vi "Main_21b.vi"() -> ()   [LabVIEW 2020]
uses:
  ENUM_Operator.ctl
  <vilib>/Utility/miscctls.llb/LVMapReplaceAction.ctl
  Cluster 21b_Monkey Data.ctl
  Map21b_Monkey Data.ctl
panel:
  out "value":i64
  out "data":string
  out "Map 2":T1
  out "total":i32
  out "itteration":i32
  out "Map":T1
  out "Answer":i32
  in  "Puzzle":string="jntc: tzrz * jmgz\nchsl: rbmj + chpp\ntmjp: rlbw + prhj\nrllz: wrgr * jplq\nbttz: hslv + jsph\npbcg: frwf - vzrg\ngfhs: 4\nsglc: 8\nrqmt: 2\nfltv: 2\nzggp: thct * ddvm\ncqdj: 8\nmslt: gsnz + blhq\nmrqj: vzvz * sdnf\nbqfd: jtlf - hmfq\npgsr: 2\nbgmj: vhqn + nnrs\nqjgh: 2\nvbwn: 2\ndftr: 2\nrphr: tnjt + vwds\nwjqp: 3\njqvb: 11\ndjcv: rtzp + ltmf\npzfg: frcg + gwdc\nsbvb: zqvr / qbtm\nfhwn: tbjd + szcc\nwdrt: 3\nhplr: gtwd * jbss\nsvgc: lddn + czqc\ncmjg: 5\nmmvj: jlbq * zdcv\nfpmz: gzjs * lwdn\ndvht: 5\ncffj: hddd + qjrz\nqcvt: rlhd * ljqt\nswqg: bvnb * wrsz\nsbmb: 7\nzmph: 3\nvjcd: qplm + fvsm\nggwg: pdfh * pjtb\nmvnq: 2\nzjgh: hqpr + bbgs\ncwzv: wfzn * dwtq\nwswt: 17\nhslp: 2\nmsct: chtt * tcvm\nfrwt: jnts * qpsz\nhnvf: pbwq + bhzw\nznsz: 2\nwfbs: 5\ndgwc: 13\ngcwt: 3\ncrhj: pznp * vcvv\npqzd: jjsc * gjnr\nqfjf: 5\ntbjd: 6\nlglj: ghnb * jdzl\ncwfj: 9\nlvqr: nlgh + nqfp\nszfs: dwdn - mcjd\ntgjh: 4\nvccz: dgcb + pqbm\nnmvr: wwvn * rsdv\ntblc: 5\nbqdv: 9\nnsft: 3\nqgvr: bpzw * mgvr\njswp: 3\nqmbr: 5\nzdcv: tlnj + qsff\nqbns: tprb / qvzt\nlftn: fmbw * jzjp\nzngc: 4\nvqzd: hjmb / dspt\nbvdt: 3\ncpqr: 2\nclhj: 5\njnnp: 2\nmjhm: 16\nzzrp: qcrs + gtbj\ntgjj: rcsj * mwmr\nrfqb: ncnl + dwgd\nzhcb: gsng + gnhq\nbbsr: 3\ndpfm: 1\nmrmp: sgvw * cmdh\ngbwd: 18\nzhcs: 3\nhnrz: 2\nwwvn: 3\nhbth: dcwg + fjrb\nbsqw: bqfd + sncr\nqzpl: fqrd * gqlh\nchtt: 10\ndtqz: 4\nsjhh: 17\nwhhm: 4\nplqr: 1\nnbmb: bvtc - ngwv\nzgcs: 2\njzjp: 2\njbfs: 11\ncchn: dpgb + ptjg\nwgvf: slhc + gmnw\ndvrf: 2\nbhjn: 2\nvrms: tczg * rhlg\nplcs: 4\ngjcs: 7\nwdfz: slwr + nqlt\ndjfv: ncjg + dbmw\ngfbs: fsrz * cqgh\nhfwt: 2\ntcpv: jgjb + vwcm\nbmjq: cpwb + nmvw\nnrwh: 4\nfqrd: 6\ndwjj: 4\npjwh: lghd / cftw\nbrwh: sbzv * cmjg\nvpts: zqnn + hflj\nvqds: vgsm + pmnv\nznlq: bqgv + dhzl\nfcls: bvbj / qpfh\nrhvf: 19\nnqnw: 3\nmlfm: 4\ngzjq: 2\nzfln: pwqd * sbmd\nqqst: jfhc * qcvt\nzprj: 3\nrvmz: ntdt + zhjb\nlqdh: cgrj + lfls\nlnbf: rtfj * ghlw\nmwdb: 9\nrclm: 12\nqpsz: 14\nqthm: rrmz * tfhq\nfmbt: twzz * wchd\nfvpj: plgp * nmtc\nqfjl: 7\nvcwg: smsr * dmdl\npttw: 8\nhwqm: znmm + mhwn\ncrnl: tdvz * fqtj\nfzwp: 5\nswfd: tscb * hdgq\nnlgh: cgdh - vdch\ndbfp: 12\npzbr: qrzt * shjp\ngmbz: chqv * lhwn\ndmjp: 2\ncjcl: 4\nljbm: 2\ntjhg: svdh * svcm\nwztf: 5\nvpmw: thmn + mtvl\nnfqr: 3\ncdzs: pntb + ncbg\nmhtc: 3\nprrj: jvvr / mpzh\nnbqf: rtvl * lqdh\nbnvv: qdgh + tght\nnqdj: 4\njmgn: 2\ngbpb: dnch * cnjf\nrgth: hmdh + vchv\nlmvn: 13\nlslm: 4\nltzd: sgwp * cmng\nfsrz: 2\nzvgp: fwhj * pzgj\nlvhs: 5\nctvm: lfvt * vmmb\ndjvv: lzjn * rclm\ntgbp: vhgv + hjch\nsjwz: 3\nqcpj: 4\nmmgz: 3\nqglw: 3\nvlgr: 2\nvcgp: hhsq + jhzd\nzhzd: 2\ntmpn: 2\nhdcz: wjhs * bbgl\ntshl: jncw - hsdj\nchps: 4\nthwz: 9\nlbzf: nfgg - bmcs\nffmm: zhjp * rbvs\nwpql: htrh / zggd\nmrmf: 19\nwnwl: jdph * fwdq\nfhfq: pgqt + fbcc\ntscb: 3\njnwm: 10\nfjhr: nftz * brss\nnsgc: 3\ndplt: 7\nwstd: ltgp + rnrf\nhztd: 5\nvnjz: brnn * bcwv\nspbn: wnjz * wnql\njhvq: 13\nzvsq: 5\nhjlp: 2\nbslw: 1\ngzzf: qwzc * wfbs\njqqv: 2\nflnz: gpfs + fnnp\nrtcg: dbfd / pfsm\ngsnz: wfts + mbnv\nnlnn: 3\njvpc: fcbt + rphr\nbdvw: jtzh * tdmd\nlzqm: 6\njtzh: 2\ntlhl: 3\nhlpt: wvfm * ssls\nmfbr: tgbp * tdtb\nwsjg: qvww + qllf\nwsdf: 15\nrtgw: 11\nfwdq: 2\njdph: mqbs * ctzc\nmrtl: 2\nhfnd: srzl * fbcb\nrgrh: 7\nnltl: 11\npgns: zffq * pbbd\nmcpb: 9\njmtj: 17\nvhfz: 8\njqmf: 7\nfrbg: 20\nqqrz: 2\ntrmp: 18\nrhng: tdmm * phjw\njmll: 12\nvqjv: 3\ntdmd: zvff + zggr\nplvh: 16\nlgfr: 3\ngncb: 2\ngvmf: 3\nrlbw: 2\nhjch: bwwq * fdsm\nnlzl: hfnd * hlrh\ntfrj: 20\nrnrf: mrgm * vwhf\nnvmm: 1\nwgmz: rhcp / rlmn\nhpbq: 3\nqjfp: 3\npjqj: 10\ndwwh: 2\nqpmt: ssjf * bmrj\njmqm: hmlj + tfcl\ngzsw: 2\nwmgn: 4\ndstw: ptbp + qnrd\nvznm: qvvs * nsft\npczb: cdfz * ghbn\nbzdz: lslm + jsdw\nhlhg: jmll + mhrz\nfgdw: wtsj * fpbt\njbbg: 3\nhfbj: 7\nrzqq: wbgw * tzdd\nlhwn: 4\npndj: 5\nszws: 4\nfrwf: jcjg + jsnv\npjfc: rtcq / zfdr\njrqq: zvsm + qzhz\nsdfq: 3\nnvmn: znlq * ssql\nqzhf: 6\nhrrn: 20\nfgjt: 11\nzhlq: 4\nnfgg: dnfh - psls\npnrq: fbzq + lbqm\nspqg: 3\nblgg: 13\ntswl: mvmn * sqbn\nqsmp: 2\ndtdb: 3\njmjp: 3\nsprd: 2\nzgmr: 3\nmwpb: pqsg + ppsm\nsjld: 2\nmvhz: nslp / wmgn\nddsm: 2\nrqnr: rlfb + nrwh\nrsnc: spth - hqfs\ndwgj: 2\ntcdj: bttz * fmnh\nvpbh: lhjn / gmcq\nnpqv: dmqt * dstn\nqmwm: jsnt + jvzj\npvtq: 9\npvhz: tstp * ltdn\nthmn: 9\nchpc: mqws * rppc\ndwdn: ndgs * nlnn\nzzpb: bvqg + pjjh\nhpfn: 5\ndfqh: fpvz - hgtm\nwnbm: 2\nczjp: 3\njcsg: 2\ndvjh: rzqq + cpvv\nwdnd: sbvw * hlrj\nlgvh: 4\nlpbr: mbww + qsmp\nmgvn: ppgd + djvv\njjlt: 20\ntzrz: 3\ncqct: hbqd / dfcj\nqzsq: 6\ndqvj: rfnc + wqzg\nhvfp: hndj + cndw\nsgqv: 19\nsvdh: 2\ncrhl: cfsr / lwhh\npwgm: 9\npgmw: 7\nccvc: qmrn + twjr\nsvsl: bmws + qjqp\njzqs: 2\nrbmj: 13\nsgwp: 9\ntlbm: fvln * jjbr\nvcwc: mrbm + rvgm\nnpzj: nbmb / cmrn\nfvzd: mfjt + gtgn\nfjbh: 2\nhtrh: cjlc * gjrf\nhlfv: zszm * pzsz\npcvb: 2\nhdbc: zwbs - rndg\nqjdc: tmjp * pmsh\nrtfb: jppl / qpft\nbdln: 2\nqqzj: vrms * nvhp\nlbrd: 5\nchlh: vsgd + gqgq\nrlpp: mnmv + wtwr\nzdzr: jnwm + cndn\nsgqc: 3\nhdgq: 3\ndsms: jmtj * svqr\nrlcp: gjcs + lnmr\nszll: 2\nbhjg: 3\nnllp: 7\nptjg: mlfm * ptbv\njfhc: 2\nqsff: 4\ngcsg: 2\njgpp: rgsh + crjw\nqghb: rqjn / bnnv\nglwr: zphr * tnzz\nvvmr: 2\ndgcb: mpqs + snbz\nbsng: sjwz + rzzm\npbcq: wgrl + ccvc\nczwl: djjt + wspf\nbslv: jlff + nvzz\npznp: 2\ndtnv: cpgw - gpvb\nsdqw: 5\ngcnq: 2\ntpnh: 2\nzmnq: qglt / tgjw\nvwnz: 5\ncmms: jgpp + rdnh\nvzwn: 2\nhqpr: 12\nqjqp: hqsp * hwrg\ndgtj: wdzt * zcnc\nnwfw: 5\nhghn: 5\nqlfm: 3\nlgtd: mcgl / vdnj\nvnct: 2\nrqjn: jnjd + hdwc\nbpql: wgvf + pmpc\nbgrc: cglv - lmmt\nljrp: 1\ntvsj: 9\nfrzb: 2\nngnc: 1\nhhsq: 2\nqwcb: 6\nljcf: 19\nwrgm: 5\nzwbs: gvjr * gztn\nbhsl: 6\nbrpr: 2\nhfrs: 5\nwdmd: 2\nvsvn: 2\nzhmz: sfld + rhng\nddvm: spnl * mwdg\nvmlh: cwzs + wnwl\ncwzs: 4\ngwfg: 4\nsnhj: gfjq + jqmf\ncwmv: 5\nppvp: rtwl * wqvr\nbqdt: bcmg + lpsh\nqpft: 3\nbcwv: mhfj + mdpd\njplq: wvld * sprd\nmwmr: 3\nnvsg: slfg + pmbv\ntgvp: 3\nfpvz: thfp * fdbs\ndcgh: 4\nbjpc: 1\njtnt: 2\nqfdm: 4\ntdlw: vbqg * tzsf\nqtnh: mrmp + blrg\nscft: 16\nbqqb: nvgh * npdt\nhcwr: 6\nczbb: 4\nfnld: 3\nqvrr: 5\npbpg: 18\nqmrh: 2\nrrcw: 14\nmcjq: 14\npzcm: 3\njlbq: 3\npslb: 3\ndqwp: jwjh - drrw\ncndg: 5\ndnfh: tmdj + wpfl\nddgd: gfbs + tfdn\njvqz: nltz / dwgj\nszvm: 10\nrlfb: 3\nllhs: scnp + fssf\nbrrr: dvgl + szvm\ngcct: brbw + hthd\nvvqj: tzwh + rzsq\njfgq: 2\nmbqg: ctvq / gvvm\nwrrt: tbnv * gwdn\nrvvm: 2\nsgpt: mstv + jpsd\nqnrd: fwsj + qthm\ntzpq: wssc * shsm\ncqhn: 13\nzjcd: qzvg * wmhn\nwqbc: 2\nfbcb: 3\nvfqs: wdjm + nrvj\nbjgz: 3\nhrld: lfcm * fqlj\ngtsh: qvvc * qpmt\nwqrr: nljh * nlgn\nsfld: 1\njmmm: bslv / plcs\nzbgv: 3\nbhbs: mqvp + qnhz\nbwcr: ghvc / bnwn\njhmn: sctd * zhgp\ncgbp: hdgc + pzfg\nrbvs: 3\nrdrc: 3\nzqjw: 2\njsvm: 7\ndtlr: 3\nvwds: cfqw * hcfh\ngrhw: zdzr + jtbs\npnlt: lvqr * tthc\nswph: tzpq - hfjh\nqrrg: 3\ndcfv: czgw * jbfs\npwdl: pnwr * wfct\nfzzh: jgrw + rnbg\nwrsz: clsz * zjtg\njnwl: 4\ntsfg: 9\ncgng: scft + cztp\ndhzl: 5\nrfnc: lrdn + cpqt\nhmtm: 1\nfrgj: tzrv + grbs\nsglr: 17\nndqw: 3\npntb: cgng + gblv\nzhgp: mmgz + qgll\nwblj: ndfv - crwz\nrzrz: hjpb * cfnc\nzgct: 8\ntrll: 4\nlbcr: wwrz + szmc\npdvm: bhhj + zjtj\ngbcd: 5\nwndj: 2\ngwcr: 16\nrqlc: 2\nmrhc: 3\nwqzg: tdfl + rwmm\nbhgc: zrcb * tfjw\ntsws: plfh * dgss\nhlsp: 3\nrstd: 16\npzsz: nzgp * qjcw\npvlj: tpjf + fjzt\nwndn: bszj * znsz\nbngj: vrns * zbgv\nwsqw: bhsr * tscd\nmtvl: svrs + lzss\ndpll: 6\nqvgj: grwn / gzpq\ntnrj: lcbc * qrrg\ntvjr: 5\nbjjz: 16\ngmsn: jzcn + cnvt\nthtw: frvh - bslw\nzjwg: 5\ntmhb: mzdb + hmss\nttpb: qwgp / vjsr\nvsgd: 6\nphwp: mglb + chpc\ntzmv: 18\nzmlh: mwfq / nzjl\nrjvg: 5\nlwdn: 7\ntdvz: zgzb * fszw\nhddd: 5\njwsw: rdml * chwp\nwwrn: 2\nhjzz: 7\ndfhb: gbpb * qwdp\nqvgl: jcsp * rjpn\nwtrb: dmrb + pbcg\nncpt: 19\nzhjb: 6\nnqlt: 5\ndjrw: pqdm + gqzj\nvncc: lnbf + dnqq\ndgpg: tgjh * csqr\nfstz: vqjs / hdff\nhrsd: 9\nvwzs: qcsr * nnlr\nmdbm: zgmc * tshn\nrqqj: spnf + ptln\nclzt: 2\nglzm: 3\ntwbs: vgsp * dcfv\nhhgj: 2\nzvsm: 7\nzsnz: vjzg + rlrf\nggwz: qfgs * hwdr\nwfgq: hlfv + tfst\nrfhb: vhcg * zjvg\nllhq: dpbg * zhcb\ntdnw: qwlz * rtfb\nllcq: 3\ngtbj: pfbd * thwz\nbjcg: lfvh + cqdj\ndttv: 12\ndsbb: crhl * pgsr\nclhw: phtz * cfrb\ntfrh: 2\nwdjm: tqrg * mrct\ndgbs: 5\nrgzs: hhzt * bsdf\nldhd: 2\nsznh: blbj + tdbt\nfgmf: 14\nsvrs: ndrr - dzdb\nzwcl: zqdm + ggcj\nchtr: lvdm * thss\nhqpj: 8\nnglb: ldnq * jfqj\nfvjr: nqdm * wcnf\nffls: 6\nmfjl: pths * zzpb\nrdhb: dvbp + pttw\nzpgb: zdzd + swrj\nzbfh: btpw * pptr\npgqt: hvrb * pnvz\ndggw: jfjv / zzzt\ndtbh: qjlz + hcnw\nnllc: mrdp + wmwg\njsnt: svdf + vnjr\nrbzr: 1\nlbdp: 3\ndwtq: wmpf * gcwt\nwgjr: qvnw + hwqm\nbrnn: 2\njszd: 7\nhcgd: tfjd * vqds\npgvl: 17\nvbzv: 2\nzsvw: 3\njncw: jswp * grqb\nqzjd: nwsw * wsgc\nbszj: vpcn - npjb\nlwcp: ddsm * dlww\nctvq: tswl * jvwq\nvdnj: 5\ngsng: 6\nzsmq: 4\ntpjf: 1\nzmbf: 3\ntfqd: vwll * bhsl\ngvpp: zqjw * lrgl\ndnpw: 3\nbfjc: 5\nvshd: 2\nrngb: sbbs * hfcw\nchpp: rbsw * chsn\nvmnp: 11\nzwbj: 4\nwvvp: zzrp * jsmg\nvssm: glsf + tjsp\npvzn: qzjb * gncr\nnnrs: grnh + rlcp\njwbl: dtpp + wngb\njsps: 2\nqncp: 5\nmtpd: 20\nvmdq: 4\nqbww: 5\nrrwf: 4\nzrcb: hmwp * tsbc\nwdjl: zdzt * rdlb\ncpvv: 2\nmpdc: pnlt - svvz\npsbc: 5\nfscs: dgnt + htrt\ncmsh: tnrj + gjpg\nsjsw: fqlv - hrnj\nsvdf: 9\nngwv: qtlj + lwqq\nsvcm: 4\nhfng: mrhc * qscw\nsdsg: nmft * bvdt\nlnld: 3\ntshn: 14\nfqbm: fgvt + lzvb\nwrsc: rtcg * ndqw\nhhzt: 5\nlmjt: 3\nsdcf: lzqw * gzzf\ntptf: 9\nqllf: hhdr * hgrc\nhsll: dzfm + tvcn\njqjq: nmlg * gnhd\nzgch: ggwz + dstc\nqhtp: gbwc * pdhv\ngfjq: nhlc * jhwm\nsjdj: cwls * wtwj\nthss: qfjf + mnwl\nmcvc: fbsn + psgw\nqzbv: mnsw + wzgz\nbdvl: wswr * tblc\nwfmj: tqgq - pwbn\ntsgh: cmbj * sdcf\nnrll: 9\nwdnm: vqzd - hnjz\nzcnc: vfdm + mwdb\nzjcr: qncp * qlqd\npvzc: chmm + tlbm\ncqvh: nrzd * ztcr\nwrvt: pzbr * dggw\ngtvf: vmsh + tvtn\nvdmw: mzjw * tvtl\ndbfd: cgdr * vhmz\nmrbm: gvzz + vdsf\ndzzn: vttd + zdhj\nlflz: mvnq * bgqp\nrlcd: 1\ncmrn: 2\ntjgd: mfjl + zjcd\nbqsd: phwp * zwfn\nnmlg: 6\nmhll: 2\nqwgm: sgcb * bwtw\nvbrn: sjrz / wjqp\nfsdh: dqvj + lsvv\nwhdh: 4\ngjnr: znrj + dptn\nnvgm: lgws * dndp\nmstv: fqrf * gsct\nztgm: gpnm - jjrt\nstzj: 4\nmsds: 5\nmgnz: 1\nctqv: vbmr * tfzv\nghzz: dtpq / mnfq\nhflj: ghqg + ctcj\njnts: rgjg + qbww\nflgb: qlfm * grcw\nslgn: 4\nljrg: 3\ndgwq: jrrs + zccc\npplh: 7\ntdfl: 3\nbmbb: fbsv * srhj\nlsvv: bgmj * hcwr\njfqj: 2\ntfcl: tptb * bgcs\nlwqq: gqlm * vlrd\nszww: 2\nszzs: 4\nfqtj: 19\npfsj: 6\nfhfh: vdvv + gzrq\nhmrt: smqq + wndn\nrnqz: fzvn * mclw\ngczf: rnqd + hfbj\nbcgd: gnpd + spgd\nsgcl: psjc / jsps\ntdbs: hcgd - fvhw\ntpgv: tdjg * gsfd\nmmll: dtpf + szll\nqzvg: 13\nrpjq: 5\nzcbc: gwcr + gmsn\nlrsg: 3\nqvnw: 5\ntlrb: tbpl + dgwc\nppsm: 7\nldpv: jrgj + dgfq\ntmdj: vbwn + rlgc\ndmgd: cbln + rgws\nsbbs: 13\nhjgm: hjvl * hwbs\nlmlz: ddll * zgjv\ngwhp: 4\nsbdl: 2\ncgrj: 2\nbwgv: 5\nfmjs: 3\nczgw: 3\ngpms: pshm + cbwl\nwlbz: 7\nldhz: 4\nrlhm: 5\nncpb: 3\nwpgl: gwhp + btsv\nnqzc: 2\nhjwf: 6\njvvr: tcpq + gvcv\nfvsm: 4\ndglb: nllp * srqm\nptln: whhm * wztf\nhnzv: lrbv + grtv\nnjvp: 14\nncbg: 9\nvzrg: 2\nncfh: 3\nwgjm: 2\ncgvc: 4\nfjnd: bjgz * qljh\njmzj: hsln * dsnc\ngrtv: 1\nfbdz: ffsm - wbwr\nlsvw: 2\ngcqf: 6\npdjr: lhrt * mjsw\nzrjf: 1\njsvj: dqcb * cclg\nhlrj: 2\nwrwg: hhcl * pfsd\nvsgs: 3\nsvqt: jdfh * wbnc\nqqzb: hhqq * zrlt\nvfqc: 4\npjtb: 2\nmrhj: 7\ngtnj: 6\nhwrg: 2\nfgsv: dvbw / pzrc\nwwrz: vdmq + mbqg\njrrs: 4\nrdvf: jcjv + mgnz\njlzd: 2\nmglp: jctm + fvpj\npnpb: 1\nwpvw: 3\nzqvr: ssnn * dwwh\ngtlb: mwcq + qdbb\nbvnb: 5\ndtjd: 2\nmtzm: bhzj * cpbj\nhcnw: 5\nnrqn: 4\nmlgm: llnj + vgwz\nrzwn: 2\nrzsq: 4\nchqv: vwss * lfgr\nvgsp: 2\nvhls: zsnz + dlnm\nclcp: 4\ndtpf: 7\nfzjv: wssd * zmph\nlppg: 10\nnjjr: sbvb * lpjg\npqlj: 5\nmglb: cpqr * gpbv\njdbd: hcgc + trmp\nblrg: msrz / mlrn\nrglm: 5\nhstd: 4\npmsp: hgnm * nbpt\nwtsj: 4\ncfrb: 2\nzmrd: pvzc * qncm\ndlpj: 2\ntqqd: 3\nhrns: zpzw * fjnd\npstz: sfcs + pzcm\nqglt: sgss * gcjt\njqnr: 7\nnnlr: 7\nzhbs: njtn + wgvm\nncch: fjrq - bjpc\nbfcn: 2\nctcj: 7\nrsdv: nrjw * mddj\ndclb: rcfh - gfhs\nhwgr: tghw + phwc\ndbwl: 2\nnvzz: 11\nntdt: vwzs + bbtf\nrccr: 2\nqdgh: 14\nndqc: qzgt + zmlh\nbmbq: hhsh * wdff\nccwq: lvrd / hnrz\nngls: 8\nqhgz: 4\nzqnn: 1\nphgr: 5\ntfhq: wqbc * tpcl\nqcmj: jbjg + hqpj\njcdp: mfrs / wgjm\nswsg: mmrl * qcmj\nprhj: 5\nbcmg: wwrn * hbvq\ndcws: 1\nzvzp: 3\nthwc: vwnz * cmgz\nchbw: cndg + sjbm\nlnrf: 2\nfnnp: tlrb * tlhl\nsrdg: 2\nspth: smzl * jbtv\nhwwc: 7\nfrnb: 3\nggcj: lcgp - gglg\ndbhh: 2\nfznq: 5\ndmtq: 8\ngsps: 8\nchtp: 5\ntffb: 2\nlztp: wqgv * tpnh\npghs: wtrb - fwmj\ntcpq: gljb / sqcs\nzzmz: vlgr * grjn\npvdq: bhqz / zpll\nhwbs: pqht + hdvs\nnzvd: zpbq + dzlz\ndstv: 13\nchts: dtdl + vpnq\nwpwm: 11\nmmrl: 9\nqqbp: cwzv * dnrj\nmslj: djfr + jszd\nlbzl: 9\nrdlb: 3\nfbsv: fpgn + mdbm\njpsd: gpvj * lptn\nwzmw: 5\nzszm: 7\ngtwd: 2\ntvtd: jmmm + rfgd\nwmpf: 2\ntgnb: svqt + wpql\nbhzj: cvmv * wgjr\nbnlh: qgvr + qrhq\nzpbq: 18\nqwqr: pvhz + trzt\nblgc: 2\njcfh: 2\npvnj: 4\nhumn: 855\nwvld: 19\ngrgv: qzpl - dbtg\nbtpw: 10\nbwtw: 9\nnthg: 2\nmddj: 3\ngfvj: 3\nbpzw: czmp * rqgt\ncpwb: 3\nnlgn: 2\nwntz: bhrv / mwvc\ntlwj: 3\nhlrh: 3\nzsdj: qfjl * rrns\nlwcm: 3\nplfh: 3\nnslp: trfg - hghn\nvcqq: 5\ncqwv: 5\nplzr: spwq + tjhg\nnqfp: 6\ndwqv: 8\ntgzm: dcgh * znpr\ngtqv: qdps + nltl\nrgjg: 2\nqqpn: 6\nwzct: vfbw + gpzw\ngdjm: 2\nwgfc: 7\nflmd: 5\nqrzt: 13\nfthr: 4\nchlt: jhbp + bnnl\nlhdb: 2\nqplg: drcm + lrtm\nrlhd: 5\nrlmn: 2\nptww: vndb + mrqj\nqjqb: 11\nzjvg: fnlz * zcbc\nqrrp: 2\ndhtd: 7\nzgmc: vgnm + ngvh\njpcs: 3\nhbvq: 4\nfvct: 13\nhhtw: 2\nwfct: fjln / fjbh\ngvjq: 8\nbhrv: vgbv * bhcb\nrtwl: 2\nvhcg: 2\nqhsv: rccr * hgvt\nrtgj: 16\nbrpn: jjlt - nfgb\nbbgs: 1\nddsq: 3\nbrhn: whlq + sznh\nbjvm: 2\ntdtc: 4\nzhpz: 2\nspwz: rjrt * jqvb\nmfgp: 2\nmhwn: 3\njhzd: 5\nmjvp: 4\ngbhw: rfqd * rhhm\ncqmn: vfvr + bqfc\nrszz: dgvf * ljbm\nwgvm: zpgb * bnvv\npsps: 5\njjvv: 2\nbpdj: 2\njvzj: 6\nvmsh: bdht / ldhd\nzjvz: whgd + gbcd\nfpbt: hgmb + djdw\nfghp: 2\nznpr: 6\nnlmw: 2\npnsw: pwbb * qcht\nhrnj: 3\ngpvj: dcvt * mpvr\nfjhf: nnsn * jngw\nsltv: 2\ndqvw: mjnp + rfnr\nllnj: bnwz + lbhv\ntptb: 11\nntqg: nqzc * lssg\ntrfg: zsft * wlbz\nswrj: gnzp * qwqr\nwvfn: wwcz - mcjn\ndwgt: 2\nltmf: 14\ntdmn: 13\nqscw: 3\nfjbm: 5\ntdbt: jchd + rtgj\ndvbw: rdtf * zccb\ntnlb: 11\nrcsj: 2\npmpc: fzjf / hfrs\nfdsm: 12\nvghh: lrpj * nglh\npmtd: 3\njchd: cnqq / gtvq\nwsvf: 2\nsvsm: zgct * fqgc\ncwpt: fbsj * wfgq\nhvrb: 5\ngzrq: 3\ntfgg: rpgm / sgvf\nplhm: ncgv * dbhh\ntbnv: 3\ncpgw: wgbc * tmhb\ntgpq: 5\nshdb: 2\nzcsn: 12\nlhsn: 3\nzgjv: nzdm + ncrp\nlcgp: jhgl * rgth\ncbwl: zjgh * lbrd\nzjbz: 5\ntrbf: 19\ntczs: czqd - twqq\nthpm: 17\nfbsj: tgjj + fqcm\nclpg: 16\nczrv: bpvp + fhfh\nqnzv: nfpp + jqjp\nwrgr: 2\ntjqq: vpmw * gbgf\nmjfs: tvsn * vfqc\nzwfn: 2\nwmzb: 10\nnltz: gwfg * lcgq\npfrm: 2\nqhfv: dzgg * nmhg\ncbbf: 3\nbvqg: hpws + cqmr\ntgzr: swbz * tjbc\nhhcl: 13\nmftw: 3\nzcgn: jfjl * msms\nsrsj: stds + fvpw\nlmdr: msml + mbgw\nvdch: 1\nbrss: sjsw * lbjm\nptbv: 4\nzhjp: mtnl + cwcb\nhsdj: cwfj * vznm\ndfpv: 2\nqjlz: 1\ngglg: 12\nrnwr: mgmh * tgnb\nhgpj: tbfn * tgtq\nhmdh: 7\nqjrz: sptw * dqvl\nrjds: 4\nqbsd: ddsq * fbvr\njjqv: vpbb * qccg\nhmvm: hjtj / mdpc\ngljb: znqs / qgms\nvpbb: dzzl + cpbb\nlbgs: 2\ngwdn: 7\npbsc: fbqr + zhwq\nvfvr: rhdz + trrq\ntlfn: 2\nblbj: tjqq + jmnf\nmcgl: zrbs + rlhm\ndmqj: qbmq / hjwf\nbqgv: dvlb * whtz\ncpbb: drfw + dmqj\nszwg: 10\nsmhb: 4\njbtv: 15\nlzvb: 12\nwwwq: bmgw * lzbl\nqlqd: wvfn + zbbp\npptr: 2\nwnfq: 16\nwdff: 17\nhcpg: 1\nvgvw: 11\nrzgg: fvbn * vccz\nqzpg: lwfh + lrtr\nznrs: 9\njnpc: blgg + gbwd\nlnlg: vmnp * vcqd\njcjg: hpdw * qjqb\nvdvv: sbmb * srvr\ngfcm: 5\nrzdv: 2\nspzn: gcqf * hnbp\nsbgb: ggsq + lfjf\ngsfd: 2\nzgbg: 4\nbhcj: nshq + lmvn\ndrrw: 4\nhcjt: 2\npzrc: 2\njfjl: 2\npctc: 6\ngggr: twgp * wpwm\nwtpb: 14\ngncr: 2\nlbnh: mctq + nlsn\nhwsh: 4\npmqv: 4\nppbd: jfqr + lzqm\ncdvf: twbs / hjlp\nnlsn: qmgp * plvh\njjlv: fmjs + bvpb\nlmmt: qwcb + hbmw\nhdwc: 13\nmqws: wmzn * sfzc\nmjsw: 12\npfjj: 2\nhngm: qzhf * jfgm\nmdpd: jvdc * nrnb\njswq: 5\nbgcs: 3\npjjh: mdbh * ctqq\nvncq: 4\njjpq: 5\nqbmq: grsz * hplr\ndzrj: cwnd + hcct\nclbs: dtbh * cbbf\nwgml: tcpv * hrpq\nmmjj: mnjh * fzqt\nffhb: 12\npwbn: pbsc + rmdr\nbtsv: 9\ngnwj: 2\nzmnl: 6\nhmwp: 2\nrdnh: qbjw + lwcp\nvnjv: mspc * sltv\nvngt: nglb / rbtf\nvccc: 2\ntrrq: ghtz + nqdj\nclsz: 2\ncwgq: msjt - ddgc\njlff: ffmz * ccfw\nrbtf: 2\njvbv: 8\nrtpm: sbdl + fvzv\nslwr: zzjt * fhwn\npjfb: 3\npqht: 17\ngjpg: zcpv * dvjq\njgjb: qrdv - njqt\nlfcm: mzmh + hmtm\nqcwp: 3\nlzwq: 3\ngqgq: 1\nmclw: vbgd + zvgp\nzrht: dtcd * swqt\nffmz: 15\njttv: 3\ncmbj: srsj + bqsd\nzrlt: 7\nrvqv: 3\nsmzl: 3\nznts: 2\ntnpc: 15\nrsff: 5\nsdhh: chlt + jvbv\ncglv: qdtw * zwbg\nppgd: tnpc + djfv\nddgr: 4\nslhp: wmzb + vshl\ntqdh: 18\nnpjb: 6\ngvjr: 7\nqwdp: tsvg / nlwp\nbvpb: 4\nqbtm: 2\nrgws: 5\nvqjs: lnpq * llhq\ntdjg: blnq + wfmj\nhlwf: ppvp + dqsf\nrtvl: mbgp - qqbl\npqzg: 5\nwfts: bzdz * dzww\nrlpt: 5\nrhdz: bmlw + gfvh\ndrtq: 3\nsjcc: stjr - jcwl\ntcvm: nbpm * swph\nwtwr: 4\nhvjz: 2\npcff: rgpp * vgwj\nwhpl: slgn * mbnm\nnnbl: 5\nznsw: 4\nhmss: fbgc + ltzd\ndpbg: 2\nfjrb: 16\nczqc: nzvd * bpsl\nsmqm: fcsb / hwwc\nzrbs: gvmf * bwmq\nwbnc: 5\nzccc: 3\nrgsh: 5\nfszm: 3\nsptw: 2\nmspc: bngj + hsgg\nwnjz: 5\ndhpc: 4\ntpdw: fnld * rvmz\ngrjb: blpq + ghgs\nlddn: mftw * sglc\nnftz: 2\ngzqc: jvzg * cltm\nqrdv: qfdm + rhjj\nlpvw: hghh + pvdq\ntzqb: 11\nzghq: bhjg * ghrv\nhnvc: 9\nnpbf: 15\nrtzp: vstr + qrhd\nchwp: mlth + pfpp\ndrfw: vbpc * brpn\nwfzn: 2\njmnt: 2\nlfls: 5\nmppr: dgpg + wrrt\npbwq: 1\nssql: 2\nwswr: prrj - pcff\ndqzd: 13\njjbt: vlln * mrhj\nwdww: nvmn * cqmn\njsnv: mtpd * lsvw\nbcbc: ngnc + mpfr\nvqfn: 10\njqjp: ptww * vhfz\nnrzd: 4\nzqgc: 9\nsgjc: jzqs * dtlr\nphrs: dsbb - jpcs\nmhql: wdrt * ljcf\ngmrn: whpl * gblj\ntppg: tdnw * rjjl\nzfdr: 2\njtdq: 5\nqplm: dplt + thtw\nblpq: brhn * hvjz\nlwfh: lgtd * tvsj\nwmhv: ppjl * srtg\nzssb: tzfp + lztp\ncpdc: gtwn * wbdm\nsrnh: mpdc + cmdp\ncmdh: 2\nfwnc: 3\nvjsr: 2\nngvh: 3\ndtpq: cffj * sjld\njvtz: 3\nzdbd: ndqc * mfgp\nvwcm: zhfb + chtr\nsdms: 3\nslhc: hmrt * sdqw\ndvbp: 11\ntmrs: 2\nswbz: jttv * hvfp\nmbcf: flwn * tpjw\nhjpb: 3\nvrns: wsdd + mhql\nmbgw: hjzz + zcsn\nlfjd: bbcm - mrcb\ncftw: 5\nsgrm: jnpm * wrdw\ndtcd: dmmd * zprj\nlmjv: swqg + qdgt\ngtgn: 1\nmbnv: 9\nccfw: pfjj + wzmw\ntptj: brwh + stzj\nwqgv: mdmr * ltbp\nrgfl: rszz + dngf\nnbpt: 2\nntpg: 2\ngnhq: 1\ncrmt: zjwg * rgrh\njjhh: rltp * vnjv\nbhqw: hztd * crmt\nzqcz: 2\njnff: lvdh * dmsb\ndspt: 3\nnzdm: qndn * ltfs\nmqbs: 6\nvgbm: 7\njnjd: nvsg + gwwt\nvsnt: zdls * hfwt\nhtqm: 3\nqdns: hnvf * qtnh\nmtft: 4\ngblj: 4\nnrjw: plts + snhf\ndnpq: sgqc * rdvf\nvlrd: pgtf + rvvm\nggrf: 3\nltbp: 5\nnrdl: 5\ngpzw: gczs + czrv\nqwlz: lgvh + zllw\nhnqg: fdqj * pghs\nsgcb: 3\nsncr: zhmz * cbcd\nbgqp: 4\ntstw: 4\nvbgd: 10\nmhht: 1\npqzw: vqsq + cfgv\nnbgc: 2\nhcfb: dpgq * cfjc\nshrc: hlpt - swfd\ngmhv: mzpd + wdww\nqjcw: 2\ngmnw: ljnd + fpcd\npths: 9\ndqcb: plvd + njsb\nqfjc: 5\nqhbl: zmbf + qhtp\nlshn: 5\nbbgl: 3\njcjv: szws * gmqd\nzdzd: 2\nvctl: wstd * htfw\njctm: mppr * szjv\nlzss: 2\nqdlt: 9\nsrlw: hwmv + rlcd\njnmb: mtzm / gjsj\nqcns: gqqb + lwvr\njlwb: fstz - mgvq\ncpqt: gczf * lhfp\ngrnh: 3\nlmgg: 17\nsdwp: pmgh * dbfj\nvjzg: 16\npphc: 3\ngrcw: 8\ngjsj: 4\ngfhp: ncpb + zsmq\nfjln: jcdp * hpwf\nvcsh: bfdc + fzwp\ngpvb: fthr * vvqj\nftjz: rpjq * qmwb\nnmhg: 2\nsbmd: 4\ncvds: pqlj + qbsj\nmqvp: pqzg * zhdn\ndvjq: vzqc - rnqz\nqbhl: 2\nfwmj: 5\nrqwf: 11\njmgz: rgbj + hcvv\nssjf: htqm * wzjp\nnlwp: 2\nzgqh: 2\npfsd: 2\nnmft: 2\nrjpn: 7\ntbzv: 5\ntjcb: 4\njtcv: 1\nthct: lbnh + sgpt\nfrcf: 4\nnbpm: 3\nzllw: 3\nsvqr: 5\ngqlm: 4\nmhfq: 6\nqmgp: 2\nhwbl: qbsd * hhgj\nqljh: bfjc + qjgh\nszfv: 2\ntdts: 17\nmzdb: vcwc * bsbw\npdfh: 7\nqzgt: znts * plzr\nszwc: wgml + nhdp\nsclh: 2\ntvcn: 8\nrhcp: mvhz + fdfl\ndqnm: 5\ncgdh: trll + gggr\nwpfl: 18\nlzjn: 7\nhdff: 2\nmgvq: 4\nnznz: 2\nrzjl: 4\npfpp: 9\nhjmb: srcv + wgpz\nqfcg: dtnv / gzjq\ngvvm: 6\ndscl: zgll * qmwm\nfhth: 4\nwmzq: 3\nrfgd: 7\ncfjc: 3\nfpcd: jlgf * sjhh\ngzpq: 5\nzdzt: 2\ntzwh: jbgr * nsgc\ntsbc: tsgh + tgzr\njjsc: 2\nzpzw: 2\ndtdl: dhpc + vsgs\ndzzl: zrjc * vnct\nrdml: 2\npbbd: zlvd + wndj\nvspw: zmrd + wzsf\ncmng: 3\ntdqs: 1\ntfdn: bvsf + wcvs\nrltp: gvpp + vcwg\nvbfb: zsvw * hbth\nlfvt: nbbg * zvzp\nhbmw: 12\ndgfq: 4\nrlnz: 2\njvzg: zcrd / wsvf\npqsg: qsrq * hjgm\nnrnb: 8\nznmm: 4\ntthc: 2\nbzjc: nrqn + qgrg\nrjrt: 2\npsls: jmnt * lcms\nwzsw: 13\nctzc: 2\ncbcd: 2\nmctq: 5\nbrlp: zggp / tmrs\nzhfb: tscr * dhgc\nnvjl: tnls + cvds\nrmfd: 8\nsbhm: 2\nplgp: nlzl + cgbp\nspjr: ssnf + clcp\ngcjt: 2\ncvzw: 11\nfqcm: 1\nlfzb: tlfn * llhs\nlrbv: zhbv + mwpb\nqwjw: hdtj - bdln\nqdlf: 3\ncrdh: 2\ntsvg: qvgl * wtpb\npnvz: 11\nqwzc: bnlh + wrvt\ngnhd: hstd * tffb\nmjnp: fdzn / sttm\nldmb: 2\nlcgq: qbhl * sbvt\njrgj: 3\nsrgd: 13\nrsgh: 3\nsrnb: 3\npgtf: 11\nrjfc: 1\nhgvt: 3\nrzlg: qgcb + mfbs\nfzjf: dzrj * rlpt\nwgzh: fjhf + mbcf\nzdls: twcp + wgzh\ncdqj: wwth + hwsh\nmbgp: ptgc * hnrp\nmpzh: 2\nfdzn: ttpb * jcsg\nsdnr: jbvw + vrdd\nlzqw: 5\ncpbj: rhvf * ntpg\nnvgh: 3\ntjbc: rvpd * brlp\ndvjc: 2\ncqll: dvjh + zwcl\njwpr: chps * qbns\nsblm: vcgp * nnbl\ntljq: 2\njtbs: lrvq * nfqr\nfnwq: sdhh * bbsr\npzmm: rzlg * sznr\nhthd: zcmj * smqm\nqpjn: tfgg - sssq\nhbqd: vsnt + ffhv\nfbvr: 3\nndfv: tfht * bcgd\nrpgm: jtnt * qlwm\nnglh: 3\nlrtr: szfv * ffmm\njngw: rzdv * czwl\nhhsh: 3\ndbtg: njvg - wrgm\nrrns: qmbr + vbzv\ntght: 11\nghlw: 7\nbqhh: 2\nbvzf: frwt - hdcz\nvnjr: 16\ngqqb: 12\nwnsn: ftqz * hsww\ngvfh: bcgt * jwff\nzhdn: tdtd / msds\nltgp: rfhb * dhwf\nsmgw: 2\nzgzb: lwzc + gzsw\nsttm: 2\nhnrp: rtsg * jsvm\ncnbl: 5\nzrff: zlgg + fbdz\nlwhh: fpmz / brpr\nvfdm: 14\nwsjb: dfwt + nlrt\nsmdv: lflz + pzmm\ncztp: rjds * rbgh\nrwgr: 12\ntgtq: zbfh - zpmp\nnfpp: wpbt + zthq\ndsbj: zhcs * pmtd\njrph: rscz * pcvb\nnjsb: 5\nhhdr: 4\nwcnf: 7\nvhqn: dpnc * dlpj\nlwzc: 5\nmdpc: 4\nqncm: 4\njtrn: zrjf + fgsv\nspmd: rnss + ncpt\ngsct: 3\ngnpd: zwsp / jffs\npsnq: fqbm + dwtm\nglpt: 2\nrrbb: rzwn * szwg\ndtpp: 4\nfmng: fmbt + mwsg\ndbfj: 4\njdww: svgc - hjbp\nzqdm: crlj * wptm\nfffz: wcht + grjw\ntnpl: jnnp * qqpn\ndztm: pvlj * tdtc\nrhlg: hhtw * nvlf\nqmwb: 6\nnpgr: ctpg - jqjq\ngwfl: bhbs + qqrz\nwmwg: gtnj * qrrp\nlrvq: 3\npvpm: wwwm / glpt\nghtz: srnb * rgfp\nwpcv: 2\nlhwl: ttwb * wpvw\ntjsp: vqmd + hvqp\ntlnp: 2\nvfbw: pvzn / hnbv\nmnfq: 2\nnwfd: 20\nhmfq: 2\nspwq: fpst * sgcl\nnshq: 6\ntpdt: 2\ngqzj: 15\nvwss: 6\ngwbq: bbzz / ttzr\ntnzz: 3\nsctd: 2\nfmrf: 7\nqzfd: zhpz * fnwq\nvhgv: lfzb / bdtl\ndnph: 2\ngtwn: fsdh + srnh\nbvbj: bmbb * jrlv\ntzfj: flgb + gtqv\nsmcr: 3\njrlv: 9\nznjt: rnmw + bpql\nzmhw: zgmr * dsdl\nbhsr: 2\ndbsw: 14\njhgl: 2\nqsbp: 7\nhgrc: 5\nljnd: gpms - lglj\nhfth: nqnw * rblm\nlrgv: vlmt * dwgt\nwdzt: 2\nblnq: mjfs * szww\ntnjt: mgvn + mjhm\ndnqq: 2\nldnq: lbdp + bjcg\nctbh: qlvw + lbzf\nssnf: cwfb * rqwf\nssls: 2\ncnvt: gfdw + hrrn\nvfjv: wnfq + rdsh\nhpwf: 2\ndmdl: 3\njbvw: dqvw * wrsc\nzvdv: 2\nfwsj: hcfm * grjb\ntfjw: 2\nfgfj: 6\npvrb: 8\nqbsj: 6\nsmrh: bpjc + mcfz\nmnmv: 3\nwgbc: 2\nnlrt: 10\nqwgp: dfpv * dsdn\nsrqm: vqfn + dpfm\nlbhv: snrr * zssb\ncrwz: flnz * fjbm\ntrct: 19\ngtvq: 2\nhwgb: wlcr * bhgc\nnrvj: 8\nqlfp: 3\nmnff: vctl / dtjd\nczqd: cqrb + vwdn\ntddg: 10\nsssq: 1\nstcr: pqzd - fgdw\nghqg: cjrg * tgnh\nfrzm: pbzz + vghh\ntqrg: 3\nmcfz: fzzh / dtdt\ngdlg: 2\nrvfj: qcns * ptnt\ntwzz: 3\nbbmm: 4\njgrw: bwcr - jnff\nbcgt: 5\nvgwj: 3\nfvwt: wvvp - psnq\nmsrz: nbgc * dglb\ndmhq: 9\ngblv: 6\nhcfh: tzqb * pvnj\nphtz: bfrr / wnbm\ndrcm: pmsp * bqqb\ncbln: 4\nggsq: 5\nmvmn: 3\npzgj: 9\nqrhq: nbqf * zgch\nfggl: 2\ncnjm: dclb / rhgt\nswhn: sdsg * ldhz\nrwtr: cwlb * qjfp\ntfjd: pbcq * jwbl\nsfnm: nmrn + nqdg\ngqlh: 18\nnzgp: 3\njqnc: mnff * drtq\nvbpc: ntqg + tgpq\nhdjv: 3\nhnbv: 2\nzsft: 7\nfvhw: fhfq * grgv\ndpgq: 4\npzph: hnvc * jpnz\nmcjd: 4\nfjrq: lhdb * ffmd\ntdmm: 3\npfqj: 15\nzgtf: 3\npmgh: wrhp + rjfc\nzphr: 3\npwqd: ljgh + gmrn\nlrtm: fffz + swsg\nqrhd: 2\nqlvw: mfwr + stbr\nsjrz: ggrf * mglp\nzzjt: 2\ntzmg: zfln * vbrn\nzbbp: 6\nnhdp: sdwp * jhvq\ncrcr: glpc * bsrl\nmcjn: 5\nfbqr: 1\nttzr: 2\njsph: lclz * ppbd\nbnwn: 3\nptgc: 2\nbgvr: sclh * sblm\nwnlf: ffls + jswq\nvstr: 5\nmrdp: gmzr * ngfj\nmzpd: njjr * bhqw\njbss: sjcc + swhn\nrtfj: 3\njppl: qdjh * zwcr\nsbzv: 5\nfjzt: 8\npplj: jwzt * tlwj\nmwcq: lmjv + fwll\nfmtl: pnjm + rsff\nphjw: 3\nroot: gvfh + njlw\nlzpd: 4\nwzsf: jnpc * jjpq\nzjtg: jwpr / znsw\nfrvh: rjmb - dtqz\njwjh: 12\nttjt: jsvj + vvmt\nfmdv: jzqn * srgd\nmgpl: jtcv + wsqw\nrtcq: qvzb / zhlq\nmpqs: mhwv * shrc\nmmgh: frzm * bzjc\nwqvr: fcnm * nthg\nwptm: 5\ntwjr: spjr + tnhq\nspnl: 2\njzqn: dppn + wntz\nfcnm: dhtd + dttv\nwzgz: 4\ngmcq: rcqp - zgcs\nqnhz: 6\nqzhc: jrcc - pmqv\ndhwf: gdlg * nddc\ncqgh: qfcg - rlwp\ndtqc: 2\ncsqr: 2\nbbcm: 10\nqjhv: 2\nwftn: dpvl + tpwr\nhslv: 4\nbhhj: 17\nltdn: 4\nmwdg: 3\nghnb: 3\nlvvz: dpgv + tdlw\ngrvq: 1\nflwn: 5\nwzjp: 11\nncgs: 5\ntpcl: fmdv + vdhh\ncfqw: 5\ndsdl: 3\nsqbn: 7\nbdtl: 2\nbmlw: 1\nvwll: lsjn + qqst\nmhfj: 1\nlsph: cqll * lbgs\nwbwr: qcpj * zgbg\nfvpw: dnpq + bhcj\nrhjj: jwsw - cbcz\ntvsn: 3\nqzdd: 5\nwvwb: 12\nbmrj: 2\nmrct: 5\nwprd: 2\nlwvr: nhnw - hcpg\ndngf: 5\nnfgb: 3\nqcnr: pslb * plcr\nhnnp: gspw - lgsw\nwrhp: 6\nrnqd: sglr * gnqp\nvzqc: pncc / bwgv\nfrbv: 10\nnhnb: 3\ntzrv: mcvc * mlgm\nzfvl: 13\npncc: tmsb + qhfv\nsnhf: rjcm + rlpp\nrrnw: rzgg + jbsd\ntbfn: 2\nbpjc: wzct + qzjd\ngmzr: 4\ncvdl: ccwq + dztm\ngtvr: 2\nzsrl: njzj * bzfw\ntrzt: 5\nrdpz: 4\nmthb: 9\nmdmr: 4\nhgnm: 5\nmfbs: 5\nfcgs: ljrg * fmrf\nncrp: lpvw * tvjr\njcsp: 3\ntzdd: 2\nlclz: 7\nhqsp: 9\ndhgc: 5\nsmqq: tfrj + pnrq\ngnqp: 2\nhgmb: wmhv - cqtg\ngbht: 2\nvpcn: fvct + hlhg\nmrcb: 3\njssr: 11\nrvpd: 2\nfzqd: 7\ngfdw: pjfb * zmhw\nhdgc: 6\nhjvl: 2\nbsbw: wnsn + qwgm\nzgrr: 2\ndpgb: pzwh + lppg\ntlnj: pbpg + pnpb\nqgll: 4\nbfdc: 1\nnqdm: 2\ngnzp: 2\nhwdr: fgjt + pqzw\ncqrb: fhth + fzqd\nnqdg: 3\nlpjg: 3\ntgnh: 3\ncgdr: 3\nghvc: bdvw - gbhw\nbsrl: tbdr * tstw\nlcms: 3\njwff: hwgb - hmvm\nghrv: 2\nfzqt: 7\nswps: pgns + pfqj\nggnl: fpzt + vdnr\nbtvd: 2\nbpvp: pjwr * dtqc\nhdvs: nqtj + wjsp\nqqbl: zzmz / wdmd\nshjp: bqdv * hzsv\nfnws: nwfd - spqg\nlvnf: rdrz + rbzr\nzwmq: gbht * qlfp\ntnhq: 1\nmlrn: 2\nhhqq: 3\nzzzt: 2\nzpmp: 3\nzgmn: 13\njcwl: jvqz + qjhv\nrcfh: zfvl * pfzw\ncsjv: 13\njtlf: 13\nqlwm: phrs * bhjn\npzlt: llzb * tsnq\nqgrg: 2\nnjqt: 4\nqgcb: djcv * jfgq\nvlmt: nvgm / dnpw\npzwh: 1\nnbbg: 3\ndbmw: frcf * wmzq\nzffq: 7\nntmd: 15\ncbcz: mcgc + hwbl\nswmf: pvpm * fmtl\nzthq: spbn * hzgq\nwlrd: 11\nszmc: 3\ndmsb: 4\ncwnd: jvpc * jhww\nzwcr: 3\ntswr: zgqh * bqdt\nqvww: cqhn * gfvq\ndfbg: 15\nmfwr: 7\ncnhc: 2\nmrsf: crdh * vqzl\nhpws: pvtq * btvd\nqnfn: clzt * dfdq\nvgsm: pdjr - wgmz\ntprb: fltv * vhls\npwbb: mthb * prwh\nsdnf: 2\nhcgc: cczv - hlqd\nfdbs: jdbd * pvdp\nddll: 2\ngpfs: 4\nrlwp: jntc + qvgj\nswqt: 4\ngrjn: rrwz + pfsj\njpcz: nznz * dgbs\njdfh: qdns + hnqg\nqdvq: sdnr / jvgj\ntlrg: 16\nnzjl: 2\nfqgc: 3\nfqlv: vqjv + wswt\nrrct: tslz * lwcm\nhcfm: tgvp * lrsg\nhzsv: 11\nrjjl: 4\ngbhl: lsph / jqqv\nqzjb: vspw * wpcv\ntsnq: lvnf * fggl\nhjwt: pstg + smdv\njvdc: 2\nfbsn: 16\nlppt: 3\nqsbh: snhj + plhm\nvcvv: lshn + tvtd\ngmqd: 2\nfrcg: 6\nctqq: 7\nwzdw: 2\nljqt: 5\njjbr: 5\nntwt: 2\nhmlj: rvqv * lmdr\ncltm: 2\nsgvf: 2\ntqgq: grhw * bjvm\ngjqf: ntzn * wfrp\nnpdt: 3\nmlth: frbg + rlnz\ndfwt: sdms * lgfr\nfqlj: 4\ntvtn: smcr * ncdz\nlfgz: fghp * zjbz\nnpmt: gfhp + szfs\nmhrz: 4\nlvrd: zjvz * bfcn\npshm: cchn * hcfb\ntwgp: 2\nblln: gwbq * bqhh\ncczv: hfng * tqqd\ndsdn: hrld - dwbl\nzbhj: 5\nchmm: vjcd - pjfc\nsgvw: lpwb + bjjz\ntdtb: 2\ndzlz: 5\nfzpn: glzm * mcpb\nqdjm: dbfp + tcdj\nhnbp: 3\nqrqw: 9\ndntn: sjsr * gcnq\npmnv: fznq * dbsw\nbbtf: qmlw * pfrm\nnqtj: rmfd + cjcl\nbvtc: zhbs / lbzl\nstds: zdbd - gjvc\nnwpz: 6\ngrqb: qjdc + npgr\nnglc: zrht + vmlh\ncmdp: ztgm * gbnp\nhjbp: zwbj * vshd\nplts: rwgr / jlzd\nqjzb: bmjq * vsvn\njgtn: 7\nntpz: wtfq * vgvw\nlrpj: 5\ndjfr: 16\nddgc: bsng * psbc\nmpvr: 2\nznrj: lhwl * bgrc\ndzww: hlsp + dwjj\ndfcj: 4\nplvd: 6\nqvvs: 7\nhfjh: 1\nsnbz: dsms + tqdh\npnwr: 2\njrcc: 12\ndptn: hdjv * wdnm\nwvfm: jrph - wnlf\nqdtw: 7\nfnlz: 2\nrtsg: 3\nfmnh: 7\nfqrf: 2\nhcct: zvwv + dzzn\nsrcv: hrns * vfqs\nqcrs: ddgd / hsnv\njmpm: tptf * drfs\nhltp: 2\nbnwz: rngb * dqwp\nvgwz: gtsh / dwqv\nfbbd: 2\nphvw: 3\nsqcs: mhtc * mlgc\ncfqs: npmt + qsbp\nchws: 3\nbsdf: 5\nglpc: 8\nlrdn: 18\nhbft: 1\nqbjw: tlrg + jqhz\nvrdd: znjt + fcls\nnhlc: 2\ntzbc: 3\nlptn: ljrp + phgr\nlgsw: qdlt + cqvh\nbdht: lrgv * wlvs\nngfj: 10\nwssc: 2\ndppn: zwmq * fsmf\nfnbj: rvbs * flmd\nwhtz: 14\ntwqq: 2\nfgsw: nwpz * nrll\nwhlq: chbw + lnlg\ngrsz: 3\nhndj: gtvf * nmvr\nzcrd: hbqp - cwjb\ndzgg: qqbp - vtms\nfpst: 2\ngwwt: 5\ndgnt: 4\ntpwr: 3\nnmvw: gdjm * vngt\nvzvz: 13\nfbgc: hdtp * pdvm\nvchv: svsl - rdpz\nsrzl: 3\ntwcp: ldwb * rstd\nmbts: gnwj * smhb\nffhv: wftn * fncq\nbnnl: mmll * nhnb\nbwmq: fpcg * dqnm\njpnz: 17\nwfrp: 4\nlbjm: 4\nfvbn: 2\nbzfw: 2\njhwm: 4\nqpfh: 3\nnvhp: zcgn - tnpl\nntbc: 4\nntzn: 2\nhtrt: 4\ngvjc: 2\njqhz: jjvv * lmgg\njlgf: jvtz + clpg\nshsm: qcwp + srlw\nndgs: tljq + rqlg\nlrgl: ltzj / frzb\njbjg: rtsn * nrdl\nwpbt: tsdv / cwmv\ndstn: 3\npfbd: qcnr / czjp\nmsms: pngq - npqv\ndpfv: 13\npbzz: 1\nlbqm: szgc + vncq\nvwhf: crcr + qdjm\nsjsr: 10\nrlrf: wlrd * dftr\ngrjw: ctvm * qcwb\nphwc: hjwt + gmhv\nbbzz: slhp * vzwn\nsvvz: 10\nrnbg: tdts * thpm\ngbgf: 5\njdhs: gbhl - pstz\nlvdh: 15\nnljh: 4\nhbqp: dbwl * qnzv\nnddc: zbhj * rglm\nghbn: 5\nhghh: tzfj + vnjz\nnpvq: 4\nfzvn: zmnl + qwjw\nffsm: shdb * tptj\ncfgv: 2\nlgws: 3\nrhzd: vgbm + cnhc\ngjvc: pwgm * lvhs\ndmmd: 4\ndwtm: clbs + qjzb\nfsmf: chts + frnb\njdzl: lpbr * gfvj\ntvtl: fszm + ngls\ntstp: 2\nwcht: znrs + rfqb\ndlww: 14\nsldj: 5\nvdhh: ctbh * dmhq\nrgbj: hsll + tnlb\nwbgw: 6\ndndp: dstw + ncwh\nwwth: 3\ndqvl: 16\ndmqt: 3\nbqfc: qpjn + dmtq\ncwfb: 5\nvgnm: srdg * qzsq\nrnss: 16\nspgd: jcfh * qplg\nvdnr: gcct * tpdw\njfgm: 7\nvtms: dscl * zqcz\nlnmr: 1\ntpjw: fjhr + fwnc\npdhv: 2\ngfvq: 3\nscnp: fgsw + wsjg\nczmp: 7\ngbnp: 8\nnhnw: svsm + dpll\nrlhz: dfhb * lmlz\nncnl: 7\nrbgh: fvzd + hbft\nvdmq: mgpl * bmfg\ntfht: 3\nwsjm: 2\nvcqd: 9\nmzjw: 2\ntfst: qpvg - wmvz\ncwls: jnwl * qvrr\nmfrs: jcbq * tmpn\nmbww: hpfn + bbmm\nhsgg: vccc * sgrm\nqmlw: zgmn * gcsg\nthfp: 2\ngvzz: mmjj * sbgb\nbpth: cwlj * dqzd\nwwwm: qnfn + jlwb\ntghw: clhw * dgtj\ngpbv: ddgr * tjcb\ngvsb: 11\ncrlj: 5\nwmnn: 2\nrdrz: mrsf + wvwb\nrjcm: 4\ndpvl: 16\nncdz: mtdc * csjv\nrscz: 17\nqvzt: 4\nzjtj: 4\nwlvs: 4\nfssf: wsjm * zrff\nwbdm: ghzz * lnrf\njbgr: 3\ntbdr: 3\nqcht: nvjl * tzbc\nmgmh: 2\nmnsw: 3\ndwbl: 5\npmsh: crhj / rqmt\nhqfs: 14\ntsnd: 2\nnmrn: dtdb * zqgc\ndsnc: mwpd + mmgh\ndlnm: hgpj * qpqs\ntzfp: cbgs + szzs\nglsf: cvzw * hssc\ncndn: 1\nvlcz: hpbq * wprd\nlsjn: zsdj + lfgz\nhzgq: 7\ndpnc: 3\nrvgm: ppng / lfjd\nptbp: dgwq * cwgq\ncrjw: fbbd * npbf\nnhsq: 14\nftqz: 4\nvshl: 3\nrzzm: jmgn * btmc\nppjl: 3\nsbvt: jqnr * wzdw\nmpfr: wgfc * dnph\nwfhg: 5\nptgz: 11\njsmg: 2\njjrt: 6\nszjv: szwc * twnf\nhssc: qzbv + bcbc\nbhqz: nglc + jmzj\ndwgd: 16\nvlln: 2\npnjm: 14\nfcsb: hfth + ctqv\ncdfz: 2\nwspf: pswj * sbhm\nrgfp: 3\nrmdr: 4\nznqs: tpgv * jmqm\nbwwq: 9\ntfzv: 7\nmtdc: hlwf + nghp\njmpz: 5\nmwfq: qrqw * zghq\ncwcb: 6\ntnls: 12\nrfqd: vbfb + rvfj\npqbm: tlnp * brrr\ngwdc: 2\nprwh: 19\ndmrb: chsl * rjvg\ncclg: 19\nzlwg: llcq * pwdl\njcbq: jtrn - dntn\nncgv: vcqq + spzn\nbmgw: gwjp * gtlb\nbrbw: blln + dfbg\nnmtc: pzph + lsvn\npfsm: 3\nzgjg: gncb * lppt\nlghd: fnws * cqwv\njzcn: 10\ndcwg: tswr + zvsq\nzvff: cmsh / hltp\nqfgs: tshl + hlpg\nqndn: tjgd - ttjt\nmlgc: 2\nstbr: 4\nfpzt: qpwm * bvzf\ncnqq: tppg / ldmb\ndrfs: 3\nvpnq: 3\ntslz: 2\nsrhj: 2\ncqmr: tzmv + nvmm\nbmbs: gtvr * sdfq\npqdm: nfnw * pgmw\ntzsf: 2\nhsnv: 2\ncmgz: tfrh * lbcr\nlhfp: 2\nzccb: glwr + tfql\nzlgg: 1\njfqr: 1\nltfs: 2\ngrwn: tfqd + vcsh\nnwsw: lvvz - npvq\njmnf: wdfz + cvdl\nvjss: czbb * ggwg\nrhhm: 3\nqpsf: 3\nlpwb: mcjq + dcws\nbhcb: 2\nlfjf: rrct * tptc\nwchd: 8\nhsww: qfnz * tpjp\ntsdv: cfqs * jmpz\nzhbv: 18\nrhgt: 5\nlcbc: rqqj * lrbm\nbmws: 5\nrlgc: 5\ntvfq: 4\nrwmm: cgvc * fcbb\nplcr: wqrr + vncc\nvhmz: fzpn + bpth\nfhrm: qhgd + tgzm\nwssd: 15\nsjvh: wblj / zhzd\nbmfg: 3\nwhgd: mhfq * rzrz\nqccg: 2\ndnch: 3\nlnpq: 4\ncqtg: 7\nlssg: 3\ndpgv: 3\nwnql: 2\nrblm: qglw * cdqj\nqpqs: 2\ndtdt: 4\nzvwv: lnld + rsgh\nzggr: rgzs * pgvl\nfwll: rhpw * mfbr\nrgpp: hnzv + rtpm\nhlqd: mjvp * zgrr\njmqs: jdhs - jjbt\nrvbs: 5\ngspw: qsbh + cmms\nnjtn: jjqv - dfqh\nqzhz: 4\nzlvd: 5\nmsjt: dvrf * hnnp\nzhwq: 6\nwgpz: mrmf * smrh\ncfsr: ldpv * jgtn\nszgc: lzwq * tpdt\ngpnm: swps - sldj\nfbzq: jmpm + jpcz\nttwb: 3\nrfnr: ffhb + rrbb\nchsn: 2\ntczg: 15\nnghp: rllz * mmvj\nctpg: thwc - gmbz\nggmh: lftn + qzpg\nrtsn: 3\nrqlg: 5\nqdps: qhgz * pczb\nmrgm: lmjt * zgtf\nlsvn: jhmn * vdmw\nqvvc: tsnd * nllc\nlvdm: 3\nbwhl: 5\nzdhj: tsfg * lhsn\ncjrg: 2\nrdtf: rnzf * zvdv\nfdfl: rsnc + sfnm\nhrpq: 3\nffmd: pjwh * bpdj\nsfzc: 5\nmbnm: 7\njfjv: ntwt * frgj\nptnt: 2\ntfql: 3\ndzdb: 1\nmfjt: 5\ncspw: 5\nldwb: pjqj + ntmd\nrrmz: wpgl * qmrh\nvttd: blgc * nwfw\ndcvt: 3\nnjlw: wwwq * pzlt\nmgvr: 7\nhlpg: zlwg + vssm\nhjtj: rbbf + rrnw\nqtlj: gvsb * qzdd\nbvsf: 8\nfqwr: ggnl + pnsw\nqcwb: 3\ncbgs: 3\ndfdq: 5\nsfcs: 5\nzwbg: hrsd + fscs\nztcr: 6\nfcbt: tdmn * nlmw\nqdbb: gjqf * dpfv\nbfrr: dvjc * jdww\nfvzv: ncgs + zgjg\nssnn: 13\nlfgr: 4\nbnnv: 2\nzggd: 2\nwrdw: 6\nmzmh: 6\nsmsr: 11\nspnf: ntpz - djrw\nslfg: fvjr * tvfq\nlrbm: 2\ntcsp: 5\nfcbb: 7\ncnjf: mslj + bmbs\nrndg: 2\nqdgt: hdbc + zsrl\npngq: phvw + gwfl\nwmhn: vjss + jrqq\ndjjt: 5\nqsrq: 2\nqvzb: gvjq * pctc\nmdbh: tczs * gvjc\ncwlb: 2\ndvgl: fhrm + mtft\nndrr: rqlc * rwtr\njwzt: 5\npsjc: 14\npvdp: 7\njbsd: chtp * qqzb\ngqjf: jmjp * chlh\ndstc: hwgr + bgvr\nwtfq: 15\nghgs: gzqc + mslt\nrqgt: tdbs + jjhh\ncndw: tzmg - rlhz\nncwh: cpdc / hcjt\nzpll: 3\ngrbs: msct + qqzj\nfszw: rrwf + qhbl\nblhq: pndj * njvp\nzgll: 2\nrhpw: 2\nsbvw: vlcz + mspq\nwjhs: tcsp + whdh\nnvlf: 5\ndqsf: fzjv - nhsq\ntbpl: 6\njsdw: plqr + jssr\nsznr: 5\npstg: dmgd * bmbq\ntmsb: rrcw * qghb\nbhzw: ntbc * bwhl\ntscr: 3\nmwvc: 2\nmnwl: 2\nmtnl: 3\ncwlj: 4\nwlcr: 8\nfwhj: 3\nltzj: dmjp * ggmh\nqmrn: 6\nsgss: jqnc + rnwr\nvbqg: jtdq + pvrb\njvwq: 2\ndgvf: zngc * qpsf\nwtwj: mhll * mbts\nfpgn: pplj + qzhc\nnjvg: 16\nszcc: wdnd + ptgz\nqcsr: 3\nllzb: vpbh * vvmr\ngwjp: 5\nlhjn: gsps * zmnq\nwjsp: 2\nrrwz: 5\nqfnz: 2\nhgtm: hngm - whlg\nwgrl: 1\nrcqp: 10\nzwsp: bdvl - sjdj\ntpjp: gqjf + lttg\nqpwm: 4\nppng: humn - swmf\ndgss: 3\nmspq: 1\nnjzj: qfjc * rqnr\ncfnc: 2\nhvqp: jmqs + cdzs\nvbmr: grvq + sgjc\ndnrj: cwpt + npzj\ntwnf: 2\nrjmb: 17\nrnzf: 5\nwngb: qdlf + fgfj\nvdsf: qzfd + rdhb\nvvmt: dstv * ftjz\nfncq: 10\nzrjc: jnmb + sjvh\nqgms: 3\npfzw: 3\nbmcs: 2\ndvlb: 2\nwcvs: cdvf * wrwg\nfbcc: 4\nnfnw: 3\nsjbm: wzsw + pplh\nmwpd: gfcm * trbf\nsrvr: 2\nfpcg: 2\ngfvh: qhsv * pphc\nhfcw: 2\nlqcc: 5\njnpm: 2\ntdtd: psps * jjlv\nhtfw: 2\ngjrf: fqwr - qdvq\nbpsl: 5\nnnsn: 2\nzmwr: 3\nrppc: 5\ngvcv: fvwt / cnbl\nqdjh: 7\ngbwc: frbv + mhht\nfvln: 2\nvgbv: 11\nzcpv: 2\nvndb: dsbj + wmnn\nvqsq: 5\njvgj: 2\nlttg: 8\nwhlg: 11\nfmbw: rgfl + rhzd\ncjlc: 4\nwsgc: 5\nfgvt: fcgs + spwz\nbpss: 7\nfdqj: 4\nwmzn: 5\nmcgc: 1\nrnmw: cqct + crnl\nrdsh: 9\nqhgd: wdjl + tsws\nbtmc: 4\ndjdw: clhj * tddg\nvmmb: 6\nmsml: 3\ngztn: rzjl + dvht\ngczs: mrtl * ncch\nhdtp: ncfh * rtgw\njhww: 2\nwsdd: 2\ncwjb: vfjv + spmd\nljgh: zjcr * fnbj\npmbv: 10\nwmvz: vmdq + sgqv\nmwsg: 13\nrbsw: 5\ndzfm: 3\nmnjh: 2\njhbp: hslp * lzpd\nqpvg: cspw * fgmf\nhwmv: 5\nhcvv: jbbg * wsdf\nstjr: fmng * tbzv\nvqmd: wsjb * rdrc\ntgjw: 2\nncjg: lqcc + wfhg\nlpsh: 5\npsgw: 7\nhpdw: 3\nvqzl: 3\nsrtg: cnjm + tdqs\npswj: chws * zmwr\nsnrr: 5\nlhrt: 11\ntscd: 3\ngzjs: 2\ntptc: 3\nzcmj: 3\ncvmv: 8\nhsln: 4\npjwr: 3\nlfvh: 2\nrbbf: stcr / smgw\nlzbl: bsqw * trct\nhdtj: 15\nhnjz: vpts + bpss\nvwdn: 2\nwwcz: 16\nmhwv: 2\njffs: 5"
  in  "Example":string="root: pppw + sjmn\ndbpl: 5\ncczh: sllz + lgvd\nzczc: 2\nptdq: humn - dvpt\ndvpt: 3\nlfqf: 4\nhumn: 5\nljgn: 2\nsjmn: drzm * dbpl\nsllz: 4\npppw: cczh / lfqf\nlgvd: ljgn * ptdq\ndrzm: hmdt - zczc\nhmdt: 32"
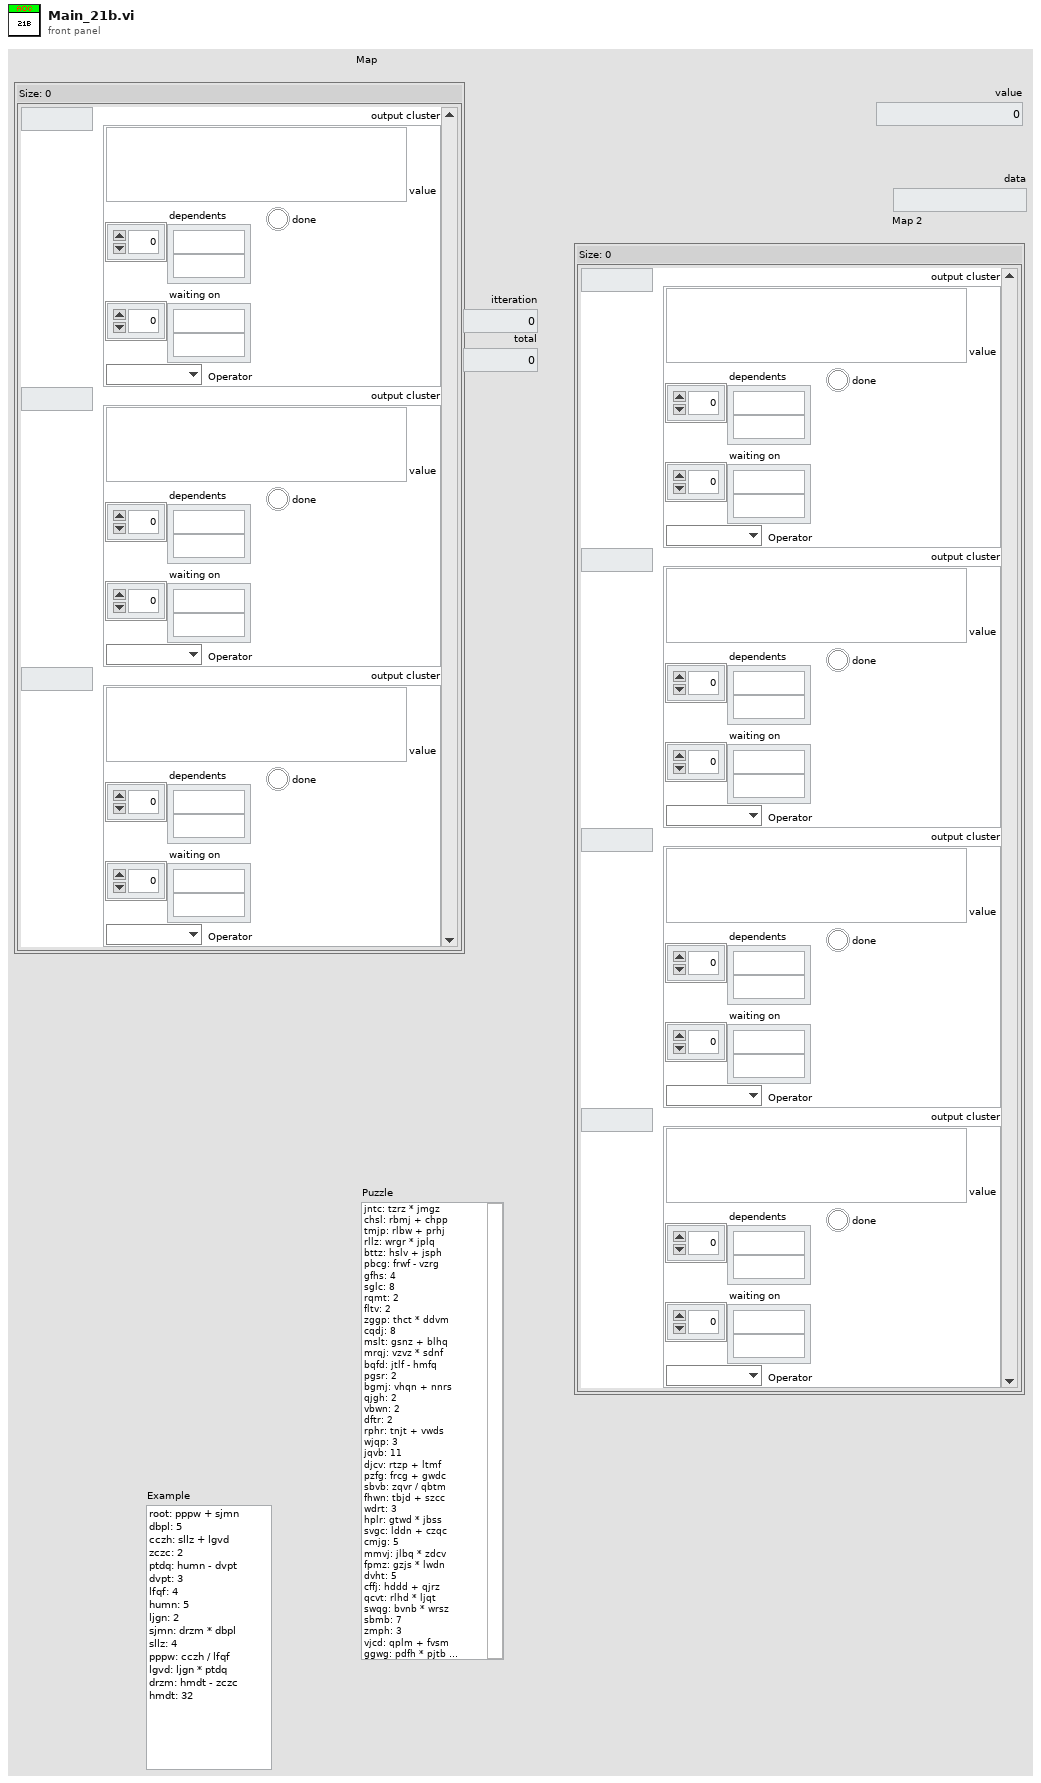
[diagram p1: front panel]
types:
  T1 = typedef "Map21b_Monkey Data.ctl" = map{string, T2}
  T2 = typedef "Cluster 21b_Monkey Data.ctl" = cluster{"done":bool, "value":string, "dependents":string[], "waiting on":string[], "Operator":T3}
  T3 = typedef "ENUM_Operator.ctl" = enum16{"Single Value", "Add", "Subtract", "Multiply", "Divide"}
  T4 = typedef "LVMapReplaceAction.ctl" = enum32{"Modify Entry only if found", "Add or Modify Entry", "Delete Entry"}
  T5 = typedef "Cluster_Monkey Data.ctl" = cluster{"done":bool, "value":i64, "dependents":string[], "waiting on":string[], "Operator":T3}
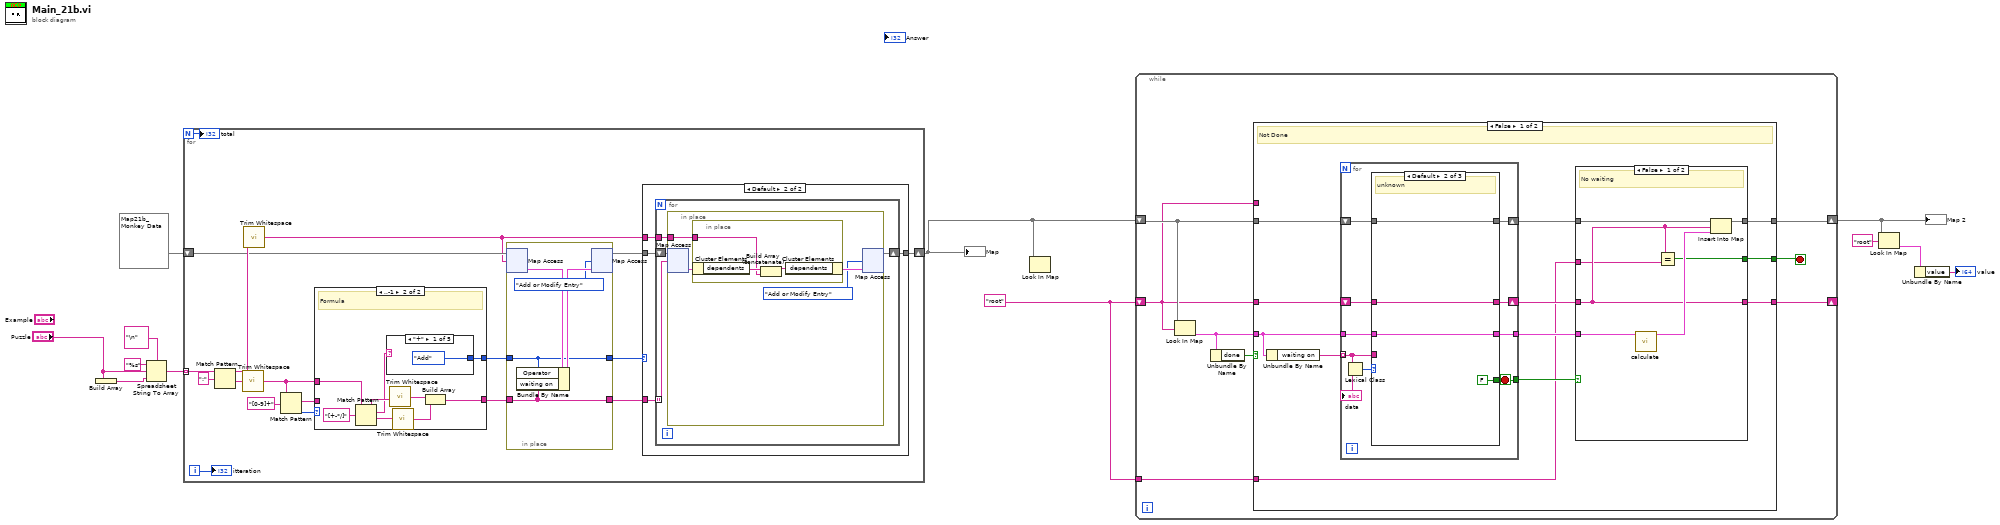
[diagram p0: block diagram]
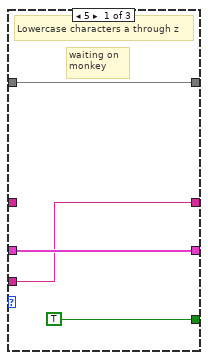
[diagram p3: hidden frame]
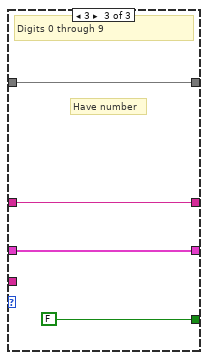
[diagram p4: hidden frame]
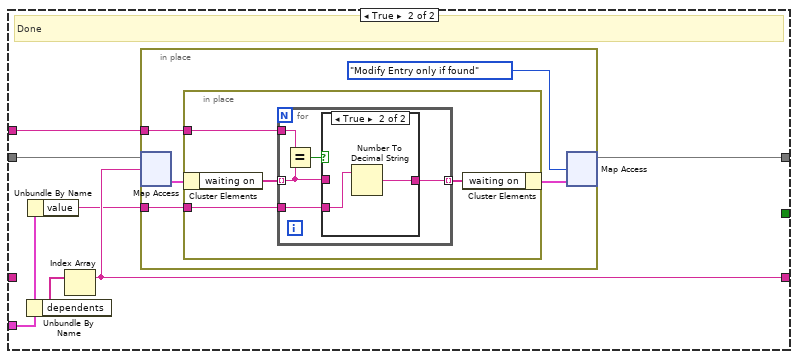
[diagram p5: hidden frame]
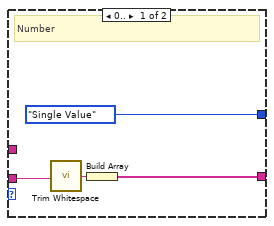
[diagram p8: hidden frame]
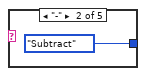
[diagram p9: hidden frame]
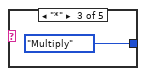
[diagram p10: hidden frame]
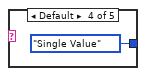
[diagram p11: hidden frame]
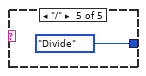
[diagram p12: hidden frame]
diagram:
  w1 = "root"
  n1 = Build Array("Puzzle") -> (w12:string[])
  n2 = Spreadsheet String To Array(delimiter (Tab)="\n", format string="%s", spreadsheet string="Puzzle", array type (2D Dbl)=w12) -> (array=w9:string[])
  n3 = for {
    N -> [w13]
    tunnel: w9 -> [w30] mode=indexing
    shift-right: [w17] -> w2
    shift-left: T1 {} -> [w23]
    i -> [w14]
    n4 = Match Pattern(string=w30, regular expression=":") -> (before substring=w27:string, after substring=w28:string)  [unwired: 1 in, 2 out]
    n5 = call <vilib>:"Trim Whitespace.vi"("string"=w28) -> ("trimmed string"=w15:string)  [unwired: 1 in]
    n6 = call <vilib>:"Trim Whitespace.vi"("string"=w27) -> ("trimmed string"=w16:string)  [unwired: 1 in]
    n7 = Match Pattern(string=w15, regular expression="[0-9]+") -> (match substring=w24:string, offset past match=w25:i32)  [unwired: 1 in, 2 out]
    n8 = case shown="..-1" w25 {
      tunnel: w24 -> [w55 _]
      tunnel: [w53 w59] -> w21
      tunnel: [ENUM_Operator."Single Value" ("Operator") w57] -> w22
      tunnel: w15 -> [_ w56]
      frame 0.. {
        # "Number"
        n9 = call <vilib>:"Trim Whitespace.vi"("string"=w55) -> ("trimmed string"=w54:string)  [unwired: 1 in]
        n10 = Build Array(w54) -> (w53:string[])
      }
      frame ..-1 {
        # "Formula"
        n11 = Match Pattern(string=w56, regular expression="[+-*/]") -> (before substring=w63:string, match substring=w58:string, after substring=w62:string)  [unwired: 1 in, 1 out]
        n12 = case shown="\"+\"" w58 {
          tunnel: [ENUM_Operator."Add" ("Operator") ENUM_Operator."Subtract" ("Operator") ENUM_Operator."Multiply" ("Operator") ENUM_Operator."Single Value" ("Operator") ENUM_Operator."Divide" ("Operator")] -> w57
          frame "+" {
          }
          frame "-" {
          }
          frame "*" {
          }
          frame Default {
          }
          frame "/" {
          }
        }
        n13 = call <vilib>:"Trim Whitespace.vi"("string"=w63) -> ("trimmed string"=w61:string)  [unwired: 1 in]
        n14 = call <vilib>:"Trim Whitespace.vi"("string"=w62) -> ("trimmed string"=w60:string)  [unwired: 1 in]
        n15 = Build Array(w61, w60) -> (w59:string[])
      }
    }
    n16 = in-place {
      in-place-border: w22 -> [w48]
      in-place-border: w21 -> [w47]
      in-place-border: [w48] -> w20
      in-place-border: [w47] -> w19
      n17 = in-place-map #1(w23, w16) -> (w51:T2)  [unwired: 1 in, 1 out]
      n18 = Bundle By Name(cluster=w51, "Operator"=w48, "waiting on"=w47) -> (w50:T2)
      n19 = in-place-map #1(w50, LVMapReplaceAction."Add or Modify Entry" ("action")) -> (w18:T1)  [unwired: 2 out]
    }
    n20 = case shown="Default" w20 {
      tunnel: w19 -> [_ w33]
      tunnel: w18 -> [w31 w35]
      tunnel: [w31 w34] -> w17
      tunnel: w16 -> [_ w32]
      frame "Single Value" {
      }
      frame Default {
        n21 = for {
          shift-right: [w36] -> w34
          shift-left: w35 -> [w39]
          tunnel: w33 -> [w38] mode=indexing
          tunnel: w32 -> [w37]
          n22 = in-place {
            in-place-border: w37 -> [w41]
            n23 = in-place-map #2(w39, w38) -> (w43:T2)  [unwired: 1 in, 1 out]
            n24 = in-place {
              in-place-border: w41 -> [w44]
              n25 = in-place-cluster #3(w43) -> ("dependents"=w46:string[])
              n26 = Build Array (concatenate)(w46, w44) -> (w45:string[])
              n27 = in-place-cluster #3("dependents"=w45) -> (w42:T2)
            }
            n28 = in-place-map #2(w42, LVMapReplaceAction."Add or Modify Entry" ("action")) -> (w36:T1)  [unwired: 2 out]
          }
        }
      }
    }
    "itteration" <- w14
    "total" <- w13
  }
  "Map" <- w2
  n29 = Look In Map(map=w2) -> ()  [unwired: 2 in, 2 out]
  n30 = while {
    shift-right: [w74] -> w6
    shift-left: w2 -> [w75]
    shift-right: [w72] -> _
    shift-left: w1 -> [w73]
    tunnel: w1 -> [w70]
    stop <- w71 stop-if-true
    n31 = Look In Map(map=w75, key=w73) -> (value=w76:T2)  [unwired: 1 in, 1 out]
    n32 = Unbundle By Name(w76) -> ("done"=w77:bool)
    n33 = case shown="False" w77 {
      tunnel: w76 -> [w88 w122]
      tunnel: w75 -> [w86 w125]
      tunnel: [w80 w123] -> w72
      tunnel: [w82 w124] -> w74
      tunnel: w73 -> [_ w121]
      tunnel: w73 -> [w87 _]
      tunnel: [w79 _] -> w71
      tunnel: w70 -> [w78 _]
      frame False {
        # "Not Done"
        n34 = Unbundle By Name(w88) -> ("waiting on"=w89:string[])
        n35 = for {
          tunnel: w89 -> [w99] mode=indexing
          shift-right: [w106] -> w83
          shift-left: w86 -> [w107]
          shift-right: [w102] -> w81
          shift-left: w87 -> [w101]
          tunnel: [w105] -> w85
          tunnel: w88 -> [w104]
          tunnel: [w103] -> w84
          stop <- w105 stop-if-true
          n36 = Lexical Class(1:w99) -> (0:w100:i16)
          n37 = case shown="Default" w100 {
            tunnel: w107 -> [w111 w115 w119]
            tunnel: [w111 w115 w119] -> w106
            tunnel: [TRUE FALSE FALSE] -> w105
            tunnel: w104 -> [w109 w114 w117]
            tunnel: [w109 w114 w117] -> w103
            tunnel: [w108 w113 w116] -> w102
            tunnel: w101 -> [_ w113 w116]
            tunnel: w99 -> [w108 _ _]
            frame 5 {
              # "waiting on \nmonkey"
              # "Lowercase characters a through z"
            }
            frame Default {
              # "unknown"
            }
            frame 3 {
              # "Have number"
              # "Digits 0 through 9"
            }
          }
          "data" <- w99
        }
        n38 = case shown="False" w85 {
          tunnel: w84 -> [w93 _]
          tunnel: w83 -> [w96 w98]
          tunnel: [w95 w98] -> w82
          tunnel: w81 -> [w92 w97]
          tunnel: [w92 w97] -> w80
          tunnel: [w91 _] -> w79
          tunnel: w78 -> [w90 _]
          frame False {
            # "No waiting"
            n39 = call "calculate.vi"("data in"=w93) -> ("data out"=w94:T5)  [unwired: 10 in]
            n40 = Equal?(x=w92, y=w90) -> (x = y?=w91:bool)
            n41 = Insert Into Map(map in=w96, key=w92, value=w94) -> (map out=w95:T1)  [unwired: 2 out]
          }
          frame True {
            # "waiting On Monkey"
          }
        }
      }
      frame True {
        # "Done"
        n42 = Unbundle By Name(w122) -> ("dependents"=w126:string[])
        n43 = Unbundle By Name(w122) -> ("value"=w120:string)
        n44 = Index Array(array=w126) -> (element=w123:string)  [unwired: 1 in]
        n45 = in-place {
          in-place-border: w121 -> [w130]
          in-place-border: w120 -> [w129]
          n46 = in-place-map #4(w125, w123) -> (w131:T2)  [unwired: 1 in, 1 out]
          n47 = in-place {
            in-place-border: w130 -> [w134]
            in-place-border: w129 -> [w133]
            n48 = in-place-cluster #5(w131) -> ("waiting on"=w135:string[])
            n49 = for {
              tunnel: w135 -> [w136] mode=indexing
              tunnel: w134 -> [w140]
              tunnel: w133 -> [w138]
              tunnel: [w137] -> w132 mode=indexing
              n50 = Equal?(x=w140, y=w136) -> (x = y?=w139:bool)
              n51 = case shown="True" w139 {
                tunnel: w138 -> [_ w143]
                tunnel: [w141 w142] -> w137
                tunnel: w136 -> [w141 _]
                frame False {
                }
                frame True {
                  n52 = Number To Decimal String(number=w143) -> (decimal integer string=w142:string)  [unwired: 1 in]
                }
              }
            }
            n53 = in-place-cluster #5("waiting on"=w132) -> (w128:T2)
          }
          n54 = in-place-map #4(w128, LVMapReplaceAction."Modify Entry only if found" ("action")) -> (w124:T1)  [unwired: 2 out]
        }
      }
    }
  }
  "Map 2" <- w6
  n55 = Look In Map(map=w6, key="root") -> (value=w4:T2)  [unwired: 1 in, 1 out]
  n56 = Unbundle By Name(w4) -> ("value"=→"value":string)
